vi "fault message.vi"(8 "error in (no error)":errorcluster, 10 "faultString":string, 11 "faultCode":i32) -> (0 "error out":errorcluster, 2 "length":i32, 3 "fault string":string)   [LabVIEW 2014]
doc: "Formats a LV error into the correct format for an XML-RPC fault response"
uses:
  struct/structMember.ctl
  SetScalarValue/IntegerAsValue.vi
  SetScalarValue/StringAsValue.vi
panel:
  in  "member (for definition)":T1
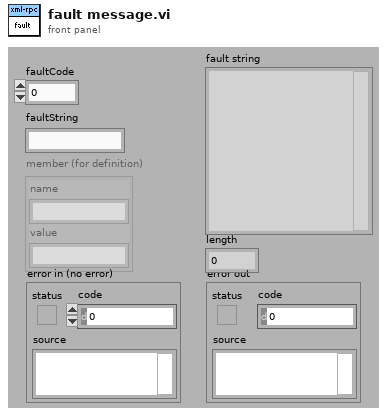
[diagram p1: front panel]
types:
  T1 = typedef "structMember.ctl" = cluster{"name":string, "value":string}
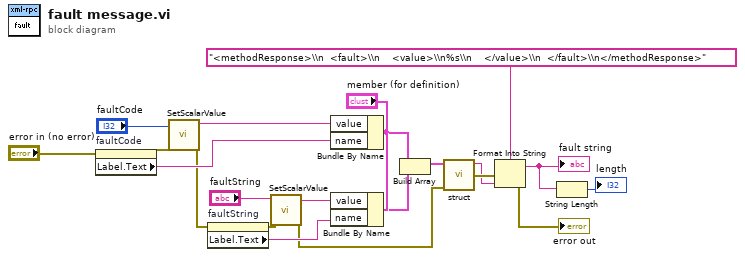
[diagram p0: block diagram]
diagram:
  n1 = property on="faultCode" class="DigNum (strict)"(error in="error in (no error)") -> (error out=w19:errorcluster, "Label.Text"=w17:string)  [unwired: 1 in, 1 out]
  n2 = call-poly "SetScalarValue.vi"("error in"=w19, "scalar value (int32)"="faultCode") -> ("error out"=w9:errorcluster, "scalar string"=w16:string)  [unwired: 8 in]
  n3 = property on="faultString" class="Str"(error in=w9) -> (error out=w18:errorcluster, "Label.Text"=w14:string)  [unwired: 1 in, 1 out]
  n4 = call-poly "SetScalarValue.vi"("error in"=w18, "scalar value (string)"="faultString") -> ("error out"=w8:errorcluster, "scalar string"=w15:string)  [unwired: 8 in]
  n5 = Bundle By Name(cluster="member (for definition)", "value"=w16, "name"=w17) -> (w12:T1)
  n6 = Bundle By Name(cluster="member (for definition)", "value"=w15, "name"=w14) -> (w11:T1)
  n7 = Build Array(w12, w11) -> (w10:T1[])
  n8 = call "struct.vi"("error in"=w8, "struct members"=w10) -> ("error out"=w6:errorcluster, "struct string"=w5:string)  [unwired: 8 in]
  n9 = Format Into String(format string="<methodResponse>\\n  <fault>\\n    <value>\\n%s\\n    </value>\\n  </fault>\\n</methodResponse>", error in=w6, w5) -> (resulting string=w3:string, error out=→"error out":errorcluster)  [unwired: 1 in]
  "fault string" <- w3
  n10 = String Length(string=w3) -> (length=→"length":i32)
